vi "MatlabTo1DArray.vi"(2 "error in (no error)":errorcluster, 3 "Array In":dbl[][](array[numeric])) -> (0 "error out":errorcluster, 1 "Array Out":dbl[](array[numeric]))   [LabVIEW 2013, in "alpD41.lvlib"]
uses:
  alpD41.lvlib
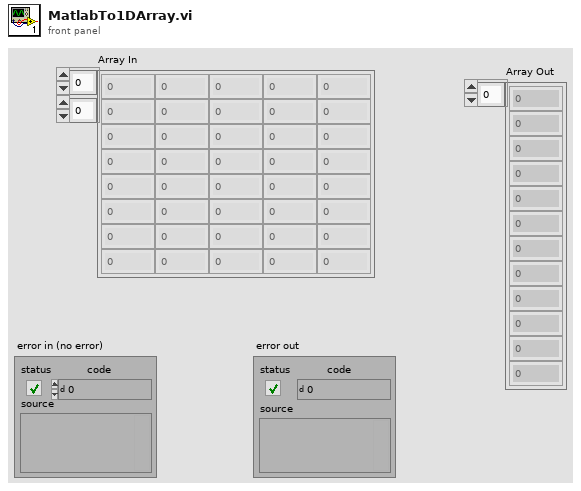
[diagram p1: front panel]
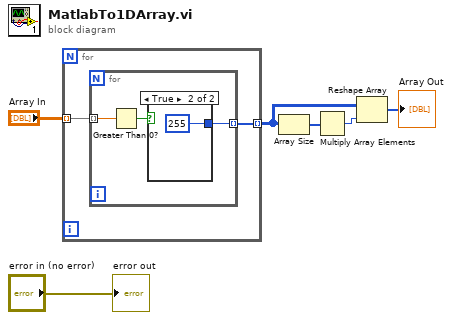
[diagram p0: block diagram]
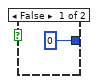
[diagram p2: hidden frame]
diagram:
  n1 = for {
    tunnel: "Array In" -> [w8] mode=indexing
    tunnel: [w7] -> w1 mode=indexing
    n2 = for {
      tunnel: w8 -> [w11] mode=indexing
      tunnel: [w9] -> w7 mode=indexing
      n3 = Greater Than 0?(x=w11) -> (x > 0?=w10:bool)
      n4 = case shown="True" w10 {
        tunnel: [u8 0 u8 255] -> w9
        frame False {
        }
        frame True {
        }
      }
    }
  }
  n5 = Array Size(array=w1) -> (size(s)=w6:i32[])
  n6 = Multiply Array Elements(1:w6) -> (0:w5:i32)
  n7 = Reshape Array(w1, w5) -> (→"Array Out":u8[])
  "error out" <- "error in (no error)"
